vi "LED Light Set Color Range.vi"() -> ()   [LabVIEW 2015]
uses:
  LED Lights Ref.ctl
  <vilib>/Rock Robotics/WPI/I2C/WPI_I2CDevRef.ctl
  <vilib>/Rock Robotics/SystemInterfaces/i2clib/i2c_bus.ctl
panel:
  out "LED Lights Ref Out":T1={"I2CDevRef"={"DevStatus"={"status"=FALSE, "code"=0, "source"=""}, "Device Address"=0, "Handle"=0, "I2C Bus"=enum."Invalid"}} {"I2CDevRef"."Device Address" format="%.0x"}
  out "error out":errorcluster
  in  "error in":errorcluster
  in  "Light ID End":u8
  in  "Light ID Start":u8
  in  "LED Lights Ref In":T1={"I2CDevRef"={"DevStatus"={"status"=FALSE, "code"=0, "source"=""}, "Device Address"=0, "Handle"=0, "I2C Bus"=enum."Invalid"}} {"I2CDevRef"."Device Address" format="%.0x"}
  in  "Color":cluster{"Red":dbl, "Green":dbl, "Blue":dbl}
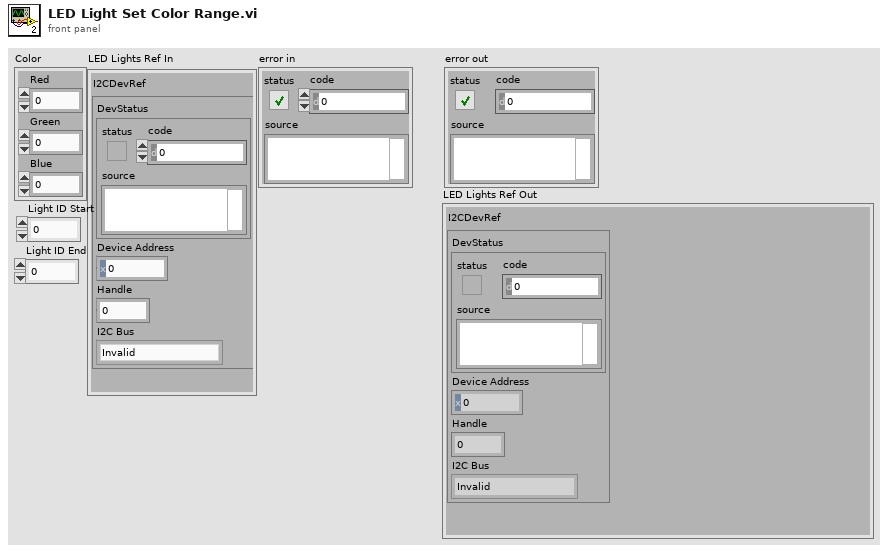
[diagram p1: front panel]
types:
  T1 = typedef "LED Lights Ref.ctl" = cluster{"I2CDevRef":T2}
  T2 = typedef "WPI_I2CDevRef.ctl" = cluster{"DevStatus":errorcluster, "Device Address":u8, "Handle":i32, "I2C Bus":T3}
  T3 = typedef "i2c_bus.ctl" = enum16{"I2C On-Board", "I2C MXP", "Invalid"}
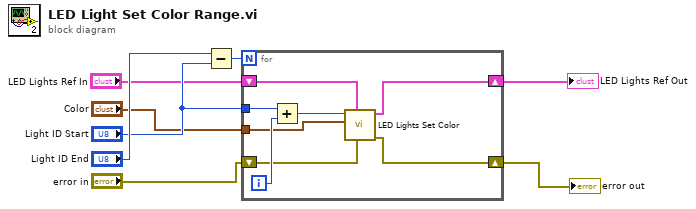
[diagram p0: block diagram]
diagram:
  n1 = Subtract(x="Light ID End", y="Light ID Start") -> (x-y=w8:u8)
  n2 = for {
    N: w8 -> [_]
    tunnel: "Light ID Start" -> [w16]
    tunnel: "Color" -> [w12]
    shift-right: [w11] -> w1
    shift-left: "LED Lights Ref In" -> [w13]
    shift-right: [w9] -> w2
    shift-left: "error in" -> [w10]
    i -> [w15]
    n3 = Add(x=w16, y=w15) -> (x+y=w14:i32)
    n4 = call "LED Lights Set Color.vi"("error in"=w10, "LED Lights Ref In"=w13, "Color"=w12, "Light ID"=w14) -> ("error out"=w9:errorcluster, "LED Lights Ref Out"=w11:T1)  [unwired: 6 in]
  }
  "error out" <- w2
  "LED Lights Ref Out" <- w1
